vi "2D-FFT with oversizing defocus complex.vi"(6 "Array in":cdb[][](array[numeric])=array256x256[65536 elements], 8 "lambda/NA":dbl, 9 "pixel size":dbl=1.0, 11 "oversize factor":i32=32) -> (0 "Array":dbl[](array[numeric]), 1 "pixel size":dbl, 3 "Array out":cdb[][](array[numeric]))   [LabVIEW 2024]
uses:
  <vilib>/Analysis/2dsp.llb/Complex FFT.vi
  <vilib>/Analysis/NI_AALPro.lvlib
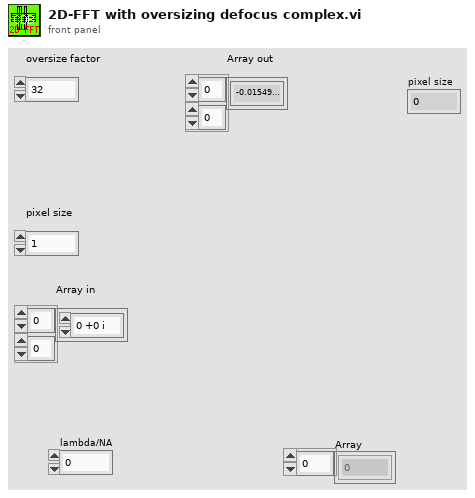
[diagram p1: front panel]
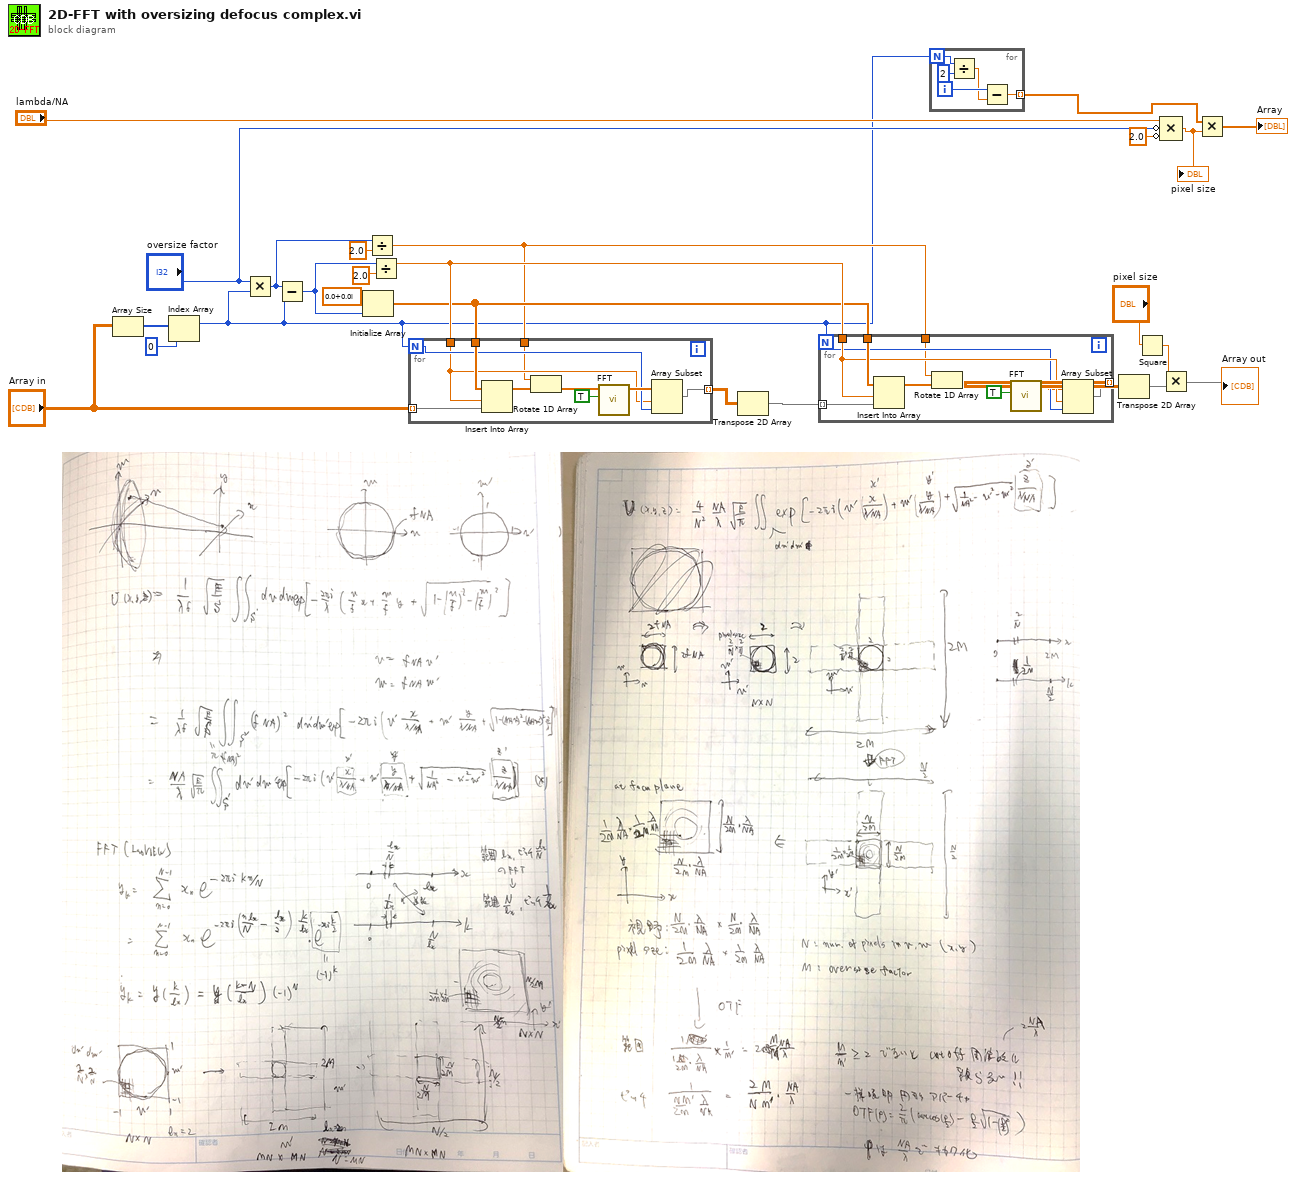
[diagram p0: block diagram]
diagram:
  n1 = Array Size(array="Array in") -> (size(s)=w12:i32[])
  n2 = Index Array(array=w12, index=0) -> (element=w4:i32)
  n3 = Multiply(x="oversize factor", y=w4) -> (x*y=w9:i32)
  n4 = Subtract(x=w9, y=w4) -> (x-y=w16:i32)
  n5 = Initialize Array(cdb 0.0+0.0i ("element"), w16) -> (w19:cdb[])
  n6 = Divide(x=w9, y=2.0) -> (x/y=w8:dbl)
  n7 = Divide(x=w16, y=2.0) -> (x/y=w20:dbl)
  n8 = for {
    N: w4 -> [w30]
    tunnel: "Array in" -> [w35] mode=indexing
    tunnel: w19 -> [w34]
    tunnel: w20 -> [w29]
    tunnel: [w28] -> w17 mode=indexing
    tunnel: w8 -> [w26]
    n9 = Insert Into Array(array=w34, index=w29, new element=w35) -> (w33:cdb[])
    n10 = Rotate 1D Array(1:w33, 2:w26) -> (0:w27:cdb[])
    n11 = call-poly <vilib>:"FFT.vi"("shift?"=TRUE, "X"=w27) -> ("FFT {X}"=w31:cdb[])  [unwired: 8 in, 1 out]
    n12 = Array Subset(array=w31, index=w29, length=w30) -> (w28:cdb[])
  }
  n13 = Transpose 2D Array(2D array=w17) -> (transposed array=w18:cdb[][])
  n14 = for {
    N: w4 -> [w40]
    tunnel: w18 -> [w45] mode=indexing
    tunnel: w19 -> [w44]
    tunnel: w20 -> [w41]
    tunnel: [w38] -> w21 mode=indexing
    tunnel: w8 -> [w36]
    n15 = Insert Into Array(array=w44, index=w41, new element=w45) -> (w43:cdb[])
    n16 = Rotate 1D Array(1:w43, 2:w36) -> (0:w37:cdb[])
    n17 = call-poly <vilib>:"FFT.vi"("shift?"=TRUE, "X"=w37) -> ("FFT {X}"=w39:cdb[])  [unwired: 8 in, 1 out]
    n18 = Array Subset(array=w39, index=w41, length=w40) -> (w38:cdb[])
  }
  n19 = for {
    N: w4 -> [w50]
    tunnel: [w46] -> w1 mode=indexing
    i -> [w48]
    n20 = Divide(x=w50, y=2) -> (x/y=w47:dbl)
    n21 = Subtract(x=w48, y=w47) -> (x-y=w46:dbl)
  }
  n22 = Transpose 2D Array(2D array=w21) -> (transposed array=w22:cdb[][])
  n23 = Square(x="pixel size") -> (x^2=w25:dbl)
  n24 = Compound Arithmetic op=MULTIPLY("lambda/NA", invert "oversize factor", invert 2.0 ("value")) -> (w2:dbl)
  "pixel size" <- w2
  n25 = Multiply(x=w25, y=w22) -> (x*y=→"Array out":cdb[][])
  n26 = Multiply(x=w1, y=w2) -> (x*y=→"Array":dbl[])
